vi "SessionControl.vi"(7 "CAN Log Path":path, 8 "error in (no error)":errorcluster, 10 "SessionEnum":enum16{"Extended", "Programming", "06"}(ring), 11 "CAN ID":T1 {"FunctionID" format="%.0x"; "ResponseID" format="%.0x"; "RequestID" format="%.0x"}) -> (0 "error out":errorcluster, 3 "Pass?":bool)   [LabVIEW 2024]
uses:
  Controls/CAN ID.ctl
panel:
  out "Data Out":u8[](array[numeric]) format="%.0x"
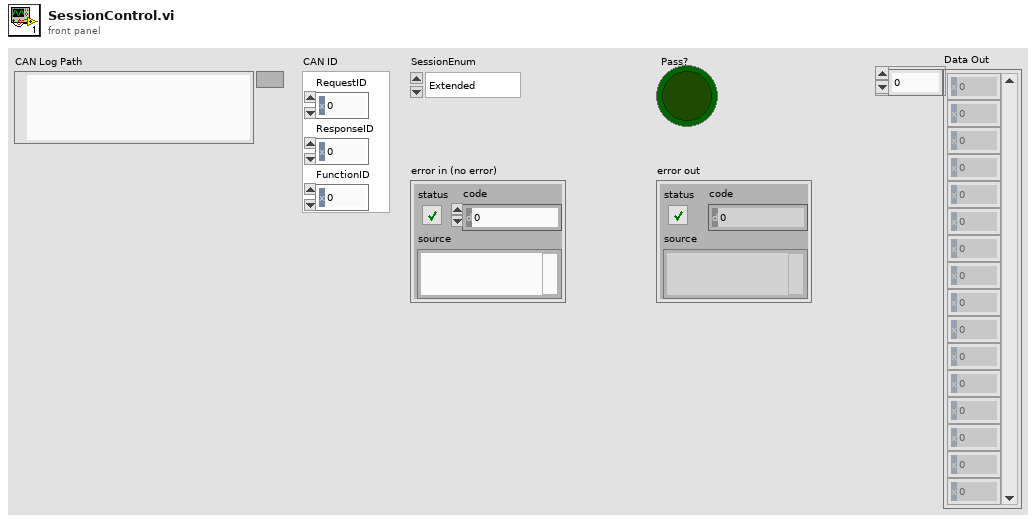
[diagram p1: front panel]
types:
  T1 = typedef "CAN ID.ctl" = cluster{"RequestID":i32, "ResponseID":i32, "FunctionID":i32}
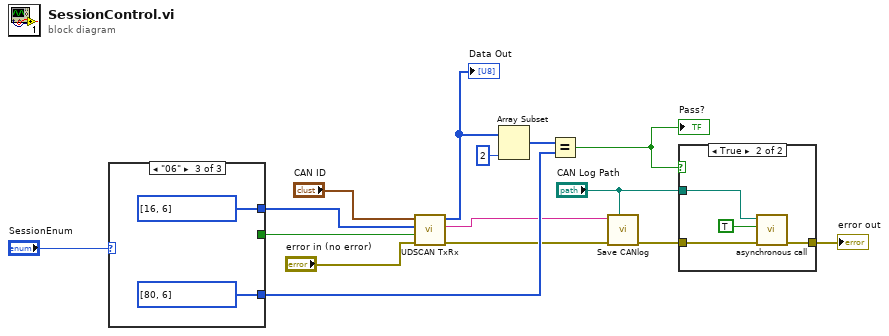
[diagram p0: block diagram]
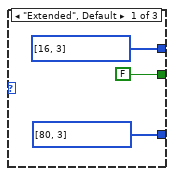
[diagram p3: hidden frame]
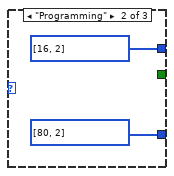
[diagram p4: hidden frame]
diagram:
  n1 = case shown="\"06\"" "SessionEnum" {
    tunnel: [FALSE ("Function?") _ _] -> w14
    tunnel: [u8[] [16, 3] ("Data In") u8[] [16, 2] ("Data In") u8[] [16, 6] ("Data In")] -> w13
    tunnel: [u8[] [80, 3] ("Data In") u8[] [80, 2] ("Data In") u8[] [80, 6] ("Data In")] -> w7
    frame "Extended", Default {
    }
    frame "Programming" {
    }
    frame "06" {
    }
  }
  n2 = call "UDSCAN TxRx.vi"("error in (no error)"="error in (no error)", "Function?"=w14, "Data In"=w13, "CAN ID"="CAN ID") -> ("error out"=w6:errorcluster, "CAN Text"=w5:string, "Data Out"=w10:u8[])  [unwired: 5 in]
  "Data Out" <- w10
  n3 = Array Subset(array=w10, length=2) -> (w8:u8[])  [unwired: 1 in]
  n4 = Equal?(x=w8, y=w7) -> (x = y?=w1:bool)
  "Pass?" <- w1
  n5 = call "Save CANlog.vi"("CAN Log Path"="CAN Log Path", "错误输入"=w6, "text"=w5) -> ("错误输出"=w4:errorcluster)  [unwired: 8 in]
  n6 = case shown="True" w1 {
    tunnel: w4 -> [w23 w27]
    tunnel: [w23 w26] -> w3
    tunnel: "CAN Log Path" -> [_ w25]
    frame False {
    }
    frame True {
      n7 = call "asynchronous call.vi"("error in (no error)"=w27, "Call？"=TRUE, "CAN Log Path"=w25) -> ("错误输出"=w26:errorcluster)  [unwired: 8 in]
    }
  }
  "error out" <- w3
